vi "9213 8Ch TC Input.vi"(1 "9213 I/O":T1={"9213 TC0"="NI 9213/TC0", "9213 TC1"="NI 9213/TC1", "9213 TC2"="NI 9213/TC2", "9213 TC3"="NI 9213/TC3", "9213 TC4"="NI 9213/TC4", "9213 TC5"="NI 9213/TC5", "9213 TC6"="NI 9213/TC6", "9213 TC7"="NI 9213/TC7", "9213 CJC"="NI 9213/CJC", "9213 Autozero"="NI 9213/Autozero"}) -> (0 "Packets":u64[](array[numeric]))   [LabVIEW 2010]
uses:
  <vilib>/eio/EIONode/EIONode.xnode
  <vilib>/rvi/eio/nirviEIOImplementation/nirviEIOImplementation.xnode
  <vilib>/rvi/eio/common/nirviEmuTemplateMethod_noerrors.vi
  <vilib>/rvi/eio/common/nirviEmuClasses.ctl
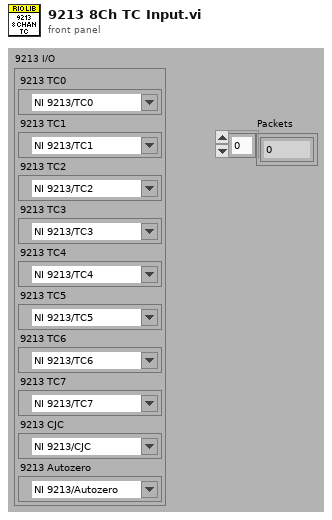
[diagram p1: front panel]
types:
  T1 = cluster{"9213 TC0":refnum<k21>, "9213 TC1":refnum<k21>, "9213 TC2":refnum<k21>, "9213 TC3":refnum<k21>, "9213 TC4":refnum<k21>, "9213 TC5":refnum<k21>, "9213 TC6":refnum<k21>, "9213 TC7":refnum<k21>, "9213 CJC":refnum<k21>, "9213 Autozero":refnum<k21>}
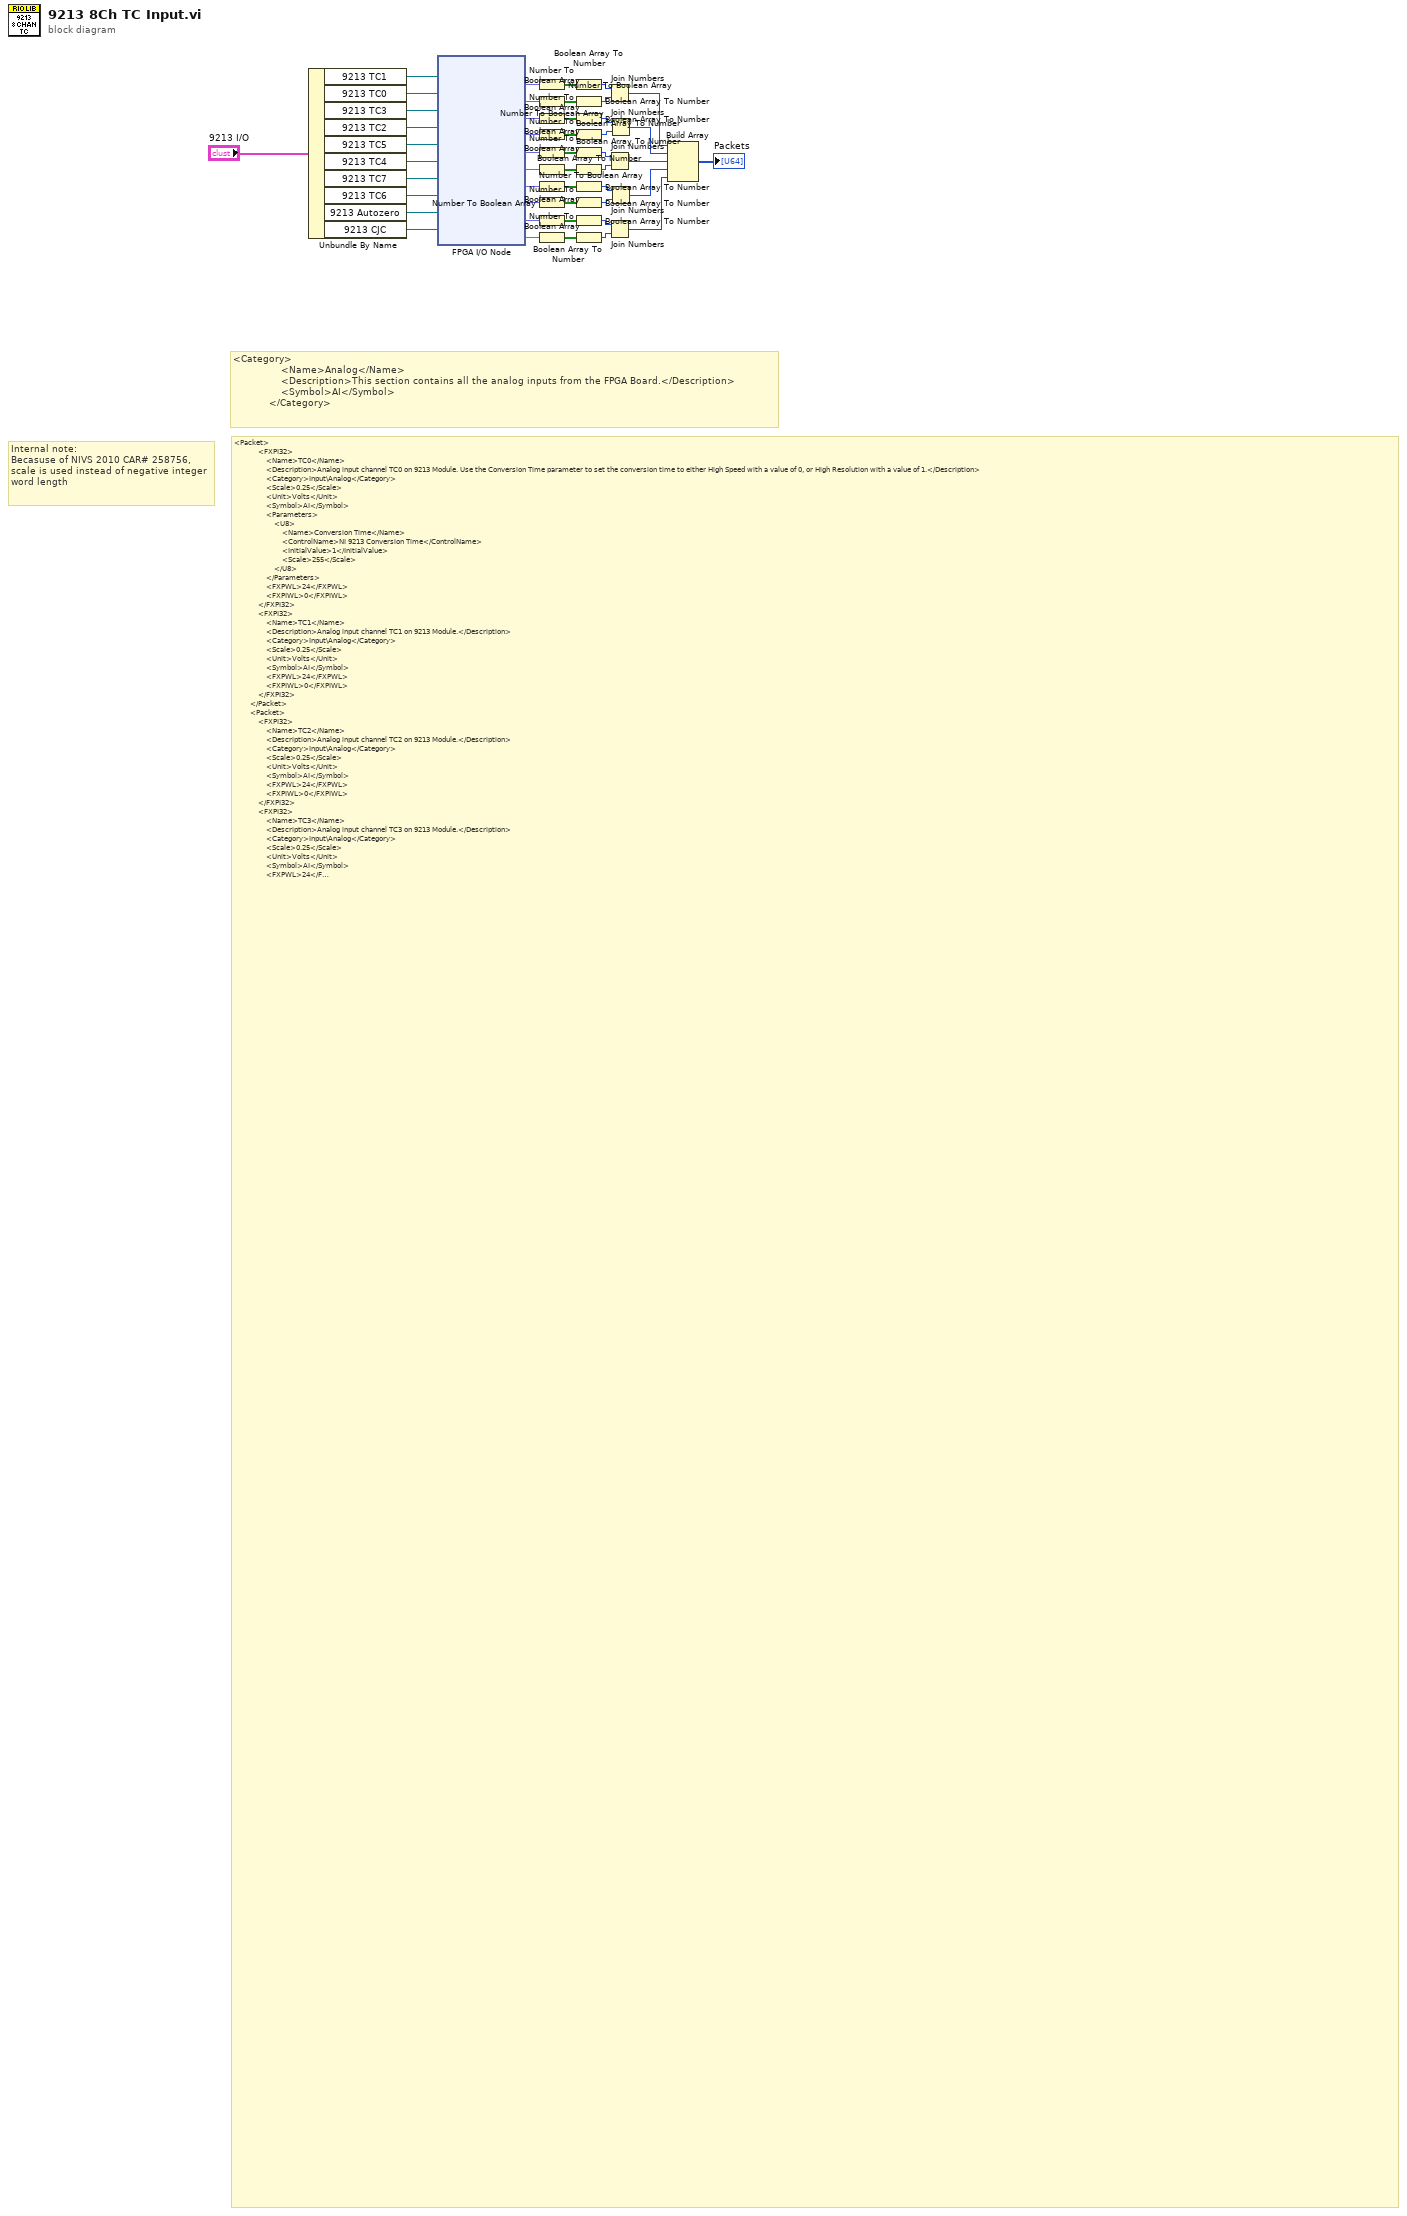
[diagram p0: block diagram]
diagram:
  # "Internal note:\nBecasuse of NIVS 2010 CAR# 258756, scale is used instead of negative integer word length"
  # "<Category>\n                <Name>Analog</Name>\n                <Description>This section contains all the analog inputs from the FPGA Board.</Description>\n                <Symbol>AI</Symbol>\n            </Category>"
  # "<Packet>\n            <FXPI32>\n                <Name>TC0</Name>\n                <Description>Analog input channel TC0 on 9213 Module. Use the Conversion Time parameter to set the conversion time to either High Speed with a value of 0, or High Resolution with a value of 1.</Description>\n                <Category>Input\\Analog</Category>\n                <Scale>0.25</Scale>\n                <Unit>Volts</Unit>\n                <Symbol>AI</Symbol>\n                <Parameters>\n                    <U8>\n                        <Name>Conversion Time</Name>\n                        <ControlName>NI 9213 Conversion Time</ControlName>\n                        <InitialValue>1</InitialValue>\n                        <Scale>255</Scale>\n                    </U8>\n                </Parameters>\n                <FXPWL>24</FXPWL>\n                <FXPIWL>0</FXPIWL>\n            </FXPI32>\n            <FXPI32>\n                <Name>TC1</Name>\n                <Description>Analog input channel TC1 on 9213 Module.</Description>\n                <Category>Input\\Analog</Category>\n                <Scale>0.25</Scale>\n                <Unit>Volts</Unit>\n                <Symbol>AI</Symbol>\n                <FXPWL>24</FXPWL>\n                <FXPIWL>0</FXPIWL>\n            </FXPI32>\n        </Packet>\n        <Packet>\n            <FXPI32>\n                <Name>TC2</Name>\n                <Description>Analog input channel TC2 on 9213 Module.</Description>\n                <Category>Input\\Analog</Category>\n                <Scale>0.25</Scale>\n                <Unit>Volts</Unit>\n                <Symbol>AI</Symbol>\n                <FXPWL>24</FXPWL>\n                <FXPIWL>0</FXPIWL>\n            </FXPI32>\n            <FXPI32>\n                <Name>TC3</Name>\n                <Description>Analog input channel TC3 on 9213 Module.</Description>\n                <Category>Input\\Analog</Category>\n                <Scale>0.25</Scale>\n                <Unit>Volts</Unit>\n                <Symbol>AI</Symbol>\n                <FXPWL>24</FXPWL>\n                <FXPIWL>0</FXPIWL>\n            </FXPI32>\n        </Packet>\n        <Packet>\n            <FXPI32>\n                <Name>TC4</Name>\n                <Description>Analog input channel TC4 on 9213 Module.</Description>\n                <Category>Input\\Analog</Category>\n                <Scale>0.25</Scale>\n                <Unit>Volts</Unit>\n                <Symbol>AI</Symbol>\n                <FXPWL>24</FXPWL>\n                <FXPIWL>0</FXPIWL>\n            </FXPI32>\n            <FXPI32>\n                <Name>TC5</Name>\n                <Description>Analog input channel TC5 on 9213 Module.</Description>\n                <Category>Input\\Analog</Category>\n                <Scale>0.25</Scale>\n                <Unit>Volts</Unit>\n                <Symbol>AI</Symbol>\n                <FXPWL>24</FXPWL>\n                <FXPIWL>0</FXPIWL>\n            </FXPI32>\n        </Packet>\n        <Packet>\n            <FXPI32>\n                <Name>TC6</Name>\n                <Description>Analog input channel TC6 on 9213 Module.</Description>\n                <Category>Input\\Analog</Category>\n                <Scale>0.25</Scale>\n                <Unit>Volts</Unit>\n                <Symbol>AI</Symbol>\n                <FXPWL>24</FXPWL>\n                <FXPIWL>0</FXPIWL>\n            </FXPI32>\n            <FXPI32>\n                <Name>TC7</Name>\n                <Description>Analog input channel TC7 on 9213 Module.</Description>\n                <Category>Input\\Analog</Category>\n                <Scale>0.25</Scale>\n                <Unit>Volts</Unit>\n                <Symbol>AI</Symbol>\n                <FXPWL>24</FXPWL>\n                <FXPIWL>0</FXPIWL>\n            </FXPI32>\n        </Packet>\n        <Packet>\n            <FXPI32>\n                <Name>CJC</Name>\n                <Description>Analog input channel CJC on 9213 Module.</Description>\n                <Category>Input\\Analog</Category>\n                <Scale>0.25</Scale>\n                <Unit>Volts</Unit>\n                <Symbol>AI</Symbol>\n                <FXPWL>24</FXPWL>\n                <FXPIWL>0</FXPIWL>\n            </FXPI32>\n            <FXPI32>\n                <Name>Autozero</Name>\n                <Description>Analog input channel Autozero on 9213 Module.</Description>\n                <Category>Input\\Analog</Category>\n                <Scale>0.25</Scale>\n                <Unit>Volts</Unit>\n                <Symbol>AI</Symbol>\n                <FXPWL>24</FXPWL>\n                <FXPIWL>0</FXPIWL>\n            </FXPI32>\n        </Packet>"
  n1 = Unbundle By Name("9213 I/O") -> ("9213 TC1"=w37:refnum<k21>, "9213 TC0"=w38:refnum<k21>, "9213 TC3"=w39:refnum<k21>, "9213 TC2"=w32:refnum<k21>, "9213 TC5"=w20:refnum<k21>, "9213 TC4"=w19:refnum<k21>, "9213 TC7"=w15:refnum<k21>, "9213 TC6"=w16:refnum<k21>, "9213 Autozero"=w17:refnum<k21>, "9213 CJC"=w18:refnum<k21>)
  n2 = xnode "FPGA I/O Node"("FPGA I/O In"=w37, "FPGA I/O In"=w38, "FPGA I/O In"=w39, "FPGA I/O In"=w32, "FPGA I/O In"=w20, "FPGA I/O In"=w19, "FPGA I/O In"=w15, "FPGA I/O In"=w16, "FPGA I/O In"=w17, "FPGA I/O In"=w18) -> ("I/O Item"=w43:fxp<+/-,24,-2>, "I/O Item"=w44:fxp<+/-,24,-2>, "I/O Item"=w29:fxp<+/-,24,-2>, "I/O Item"=w31:fxp<+/-,24,-2>, "I/O Item"=w23:fxp<+/-,24,-2>, "I/O Item"=w22:fxp<+/-,24,-2>, "I/O Item"=w6:fxp<+/-,24,-2>, "I/O Item"=w5:fxp<+/-,24,-2>, "I/O Item"=w4:fxp<+/-,24,-2>, "I/O Item"=w3:fxp<+/-,24,-2>)  [unwired: 10 out]
  n3 = Number To Boolean Array(number=w43) -> (Boolean array=w40:bool[])
  n4 = Number To Boolean Array(number=w44) -> (Boolean array=w41:bool[])
  n5 = Number To Boolean Array(number=w29) -> (Boolean array=w28:bool[])
  n6 = Number To Boolean Array(number=w31) -> (Boolean array=w42:bool[])
  n7 = Number To Boolean Array(number=w23) -> (Boolean array=w27:bool[])
  n8 = Number To Boolean Array(number=w22) -> (Boolean array=w26:bool[])
  n9 = Number To Boolean Array(number=w6) -> (Boolean array=w10:bool[])
  n10 = Number To Boolean Array(number=w5) -> (Boolean array=w8:bool[])
  n11 = Number To Boolean Array(number=w4) -> (Boolean array=w11:bool[])
  n12 = Number To Boolean Array(number=w3) -> (Boolean array=w12:bool[])
  n13 = Boolean Array To Number(Boolean array=w40) -> (number=w45:u32)
  n14 = Boolean Array To Number(Boolean array=w41) -> (number=w46:u32)
  n15 = Boolean Array To Number(Boolean array=w28) -> (number=w30:u32)
  n16 = Boolean Array To Number(Boolean array=w42) -> (number=w47:u32)
  n17 = Boolean Array To Number(Boolean array=w27) -> (number=w25:u32)
  n18 = Boolean Array To Number(Boolean array=w26) -> (number=w24:u32)
  n19 = Boolean Array To Number(Boolean array=w10) -> (number=w9:u32)
  n20 = Boolean Array To Number(Boolean array=w8) -> (number=w7:u32)
  n21 = Boolean Array To Number(Boolean array=w11) -> (number=w13:u32)
  n22 = Boolean Array To Number(Boolean array=w12) -> (number=w14:u32)
  n23 = Join Numbers(hi=w45, lo=w46) -> ((hi.lo)=w35:u64)
  n24 = Join Numbers(hi=w25, lo=w24) -> ((hi.lo)=w21:u64)
  n25 = Join Numbers(hi=w13, lo=w14) -> ((hi.lo)=w2:u64)
  n26 = Join Numbers(hi=w30, lo=w47) -> ((hi.lo)=w36:u64)
  n27 = Join Numbers(hi=w9, lo=w7) -> ((hi.lo)=w1:u64)
  n28 = Build Array(w35, w36, w21, w1, w2) -> (→"Packets":u64[])
